vi "Remove Elements from Linker Info Array.vi"(9 "elements to remove":i32[](array[numeric]), 10 "Linker Info":T1(array[cluster])) -> (2 "Linker Info out":T1(array[cluster]))   [LabVIEW 2020]
uses:
  <vilib>/addons/_JKI.lib/_jki_lib_array.llb/X in Y (I32)__jki_lib_array.vi
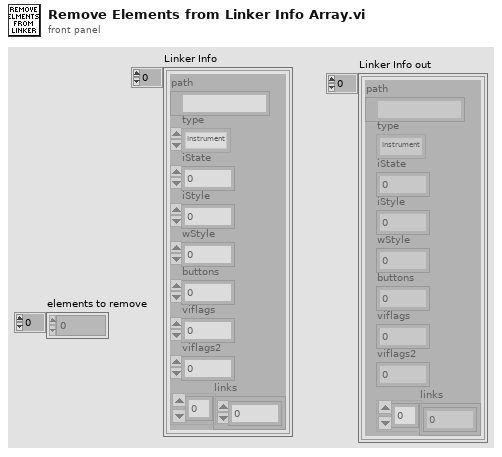
[diagram p1: front panel]
types:
  T1 = cluster{"path":path, "type":enum32{"Instrument", "Control", "CIN", "External subroutine", "Shared library", "Run-time menu", "Help file", "Palette menu"}, "iState":u32, "iStyle":u16, "wStyle":u16, "buttons":u16, "viflags":u32, "viflags2":u32, "links":u32[]}[]
  T2 = cluster{"path":path, "type":enum32{"Instrument", "Control", "CIN", "External subroutine", "Shared library", "Run-time menu", "Help file", "Palette menu"}, "iState":u32, "iStyle":u16, "wStyle":u16, "buttons":u16, "viflags":u32, "viflags2":u32, "links":u32[]}
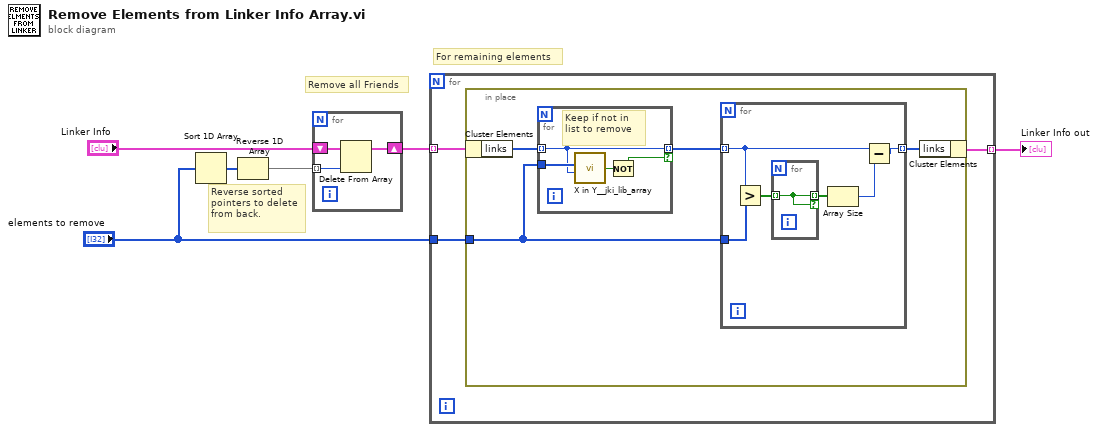
[diagram p0: block diagram]
diagram:
  # "For remaining elements"
  # "Reverse sorted pointers to delete from back."
  # "Remove all Friends"
  n1 = Sort 1D Array(array="elements to remove") -> (sorted array=w6:i32[])
  n2 = Reverse 1D Array(array=w6) -> (reversed array=w1:i32[])
  n3 = for {
    tunnel: w1 -> [w8] mode=indexing
    shift-right: [w7] -> w2
    shift-left: "Linker Info" -> [w9]
    n4 = Delete From Array(array=w9, index=w8) -> (array with subset deleted=w7:T1)  [unwired: 1 in, 1 out]
  }
  n5 = for {
    tunnel: w2 -> [w12] mode=indexing
    tunnel: "elements to remove" -> [w11]
    tunnel: [w10] -> w5 mode=indexing
    n6 = in-place {
      in-place-border: w11 -> [w14]
      n7 = in-place-cluster #1(w12) -> ("links"=w16:u32[])
      n8 = for {
        tunnel: w16 -> [w25] mode=indexing
        tunnel: w14 -> [w27]
        tunnel: [w25] -> w15 mode=indexing if=w24
        # "Keep if not in list to remove"
        n9 = call-poly <vilib>:"X in Y__jki_lib_array.vi"("array"=w27, "element"=w25) -> ("element in array?"=w26:bool)  [unwired: 5 in]
        n10 = Not(x=w26) -> (.not. x?=w24:bool)
      }
      n11 = for {
        tunnel: w15 -> [w18] mode=indexing
        tunnel: w14 -> [w22]
        tunnel: [w17] -> w13 mode=indexing
        n12 = Greater?(x=w18, y=w22) -> (0:w21:bool[])
        n13 = for {
          tunnel: [w23] -> w20 mode=indexing if=w23
          tunnel: w21 -> [w23] mode=indexing
        }
        n14 = Array Size(array=w20) -> (size(s)=w19:i32)
        n15 = Subtract(x=w18, y=w19) -> (x-y=w17:u32)
      }
      n16 = in-place-cluster #1("links"=w13) -> (w10:T2)
    }
  }
  "Linker Info out" <- w5
